vi "SMD7615 UDP Close.vi"(8 "error in (no error)":errorcluster, 10 "IP":string="192.168.1.30", 11 "connection ID in":refnum<k16>) -> (0 "error out":errorcluster, 3 "connection ID out":refnum<k16>)   [LabVIEW 2016, in "SMD-7615.lvlib" / "eSCL.lvlib"]
uses:
  eSCL.lvlib
panel:
  out "Status 2":string
  out "Status":string
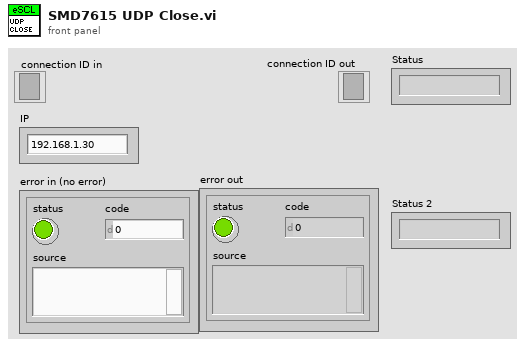
[diagram p1: front panel]
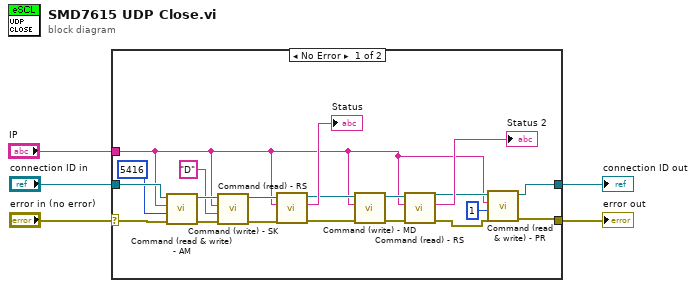
[diagram p0: block diagram]
diagram:
  n1 = case shown="No Error" "error in (no error)" {
    selector: "error in (no error)" -> [w19 w26]
    tunnel: "connection ID in" -> [w18 w27]
    tunnel: [w10 w27] -> w3
    tunnel: [w9 w26] -> w2
    tunnel: "IP" -> [w6 _]
    frame No Error {
      n2 = call "Command (read & write) - AM.vi"("error in (no error)"=w19, "Max. Acceleration"=5416, "IP"=w6, "connection ID in"=w18) -> ("error out"=w15:errorcluster, "connection ID out"=w16:refnum<k16>)  [unwired: 6 in]
      n3 = call "Command (write) - SK.vi"("error in (no error)"=w15, "Parameter"="D", "IP"=w6, "connection ID in"=w16) -> ("error out"=w12:errorcluster, "connection ID out"=w13:refnum<k16>)  [unwired: 6 in]
      n4 = call "Command (read) - RS.vi"("error in (no error)"=w12, "IP"=w6, "connection ID in"=w13) -> ("error out"=w21:errorcluster, "Status"=→"Status":string, "connection ID out"=w20:refnum<k16>)  [unwired: 6 in]
      n5 = call "Command (write) - MD.vi"("error in (no error)"=w21, "IP"=w6, "connection ID in"=w20) -> ("error out"=w22:errorcluster, "connection ID out"=w23:refnum<k16>)  [unwired: 7 in]
      n6 = call "Command (read) - RS.vi"("error in (no error)"=w22, "IP"=w6, "connection ID in"=w23) -> ("error out"=w8:errorcluster, "Status"=→"Status 2":string, "connection ID out"=w11:refnum<k16>)  [unwired: 6 in]
      n7 = call "Command (read & write) - PR.vi"("error in (no error)"=w8, "Protocol Setting"=1, "IP"=w6, "connection ID in"=w11) -> ("error out"=w9:errorcluster, "connection ID out"=w10:refnum<k16>)  [unwired: 5 in, 1 out]
    }
    frame Error {
    }
  }
  "connection ID out" <- w3
  "error out" <- w2
